vi "User_Manage.vi"() -> ()   [LabVIEW 2020]
panel:
  in  "User List":i32(listbox)
  # "用户管理"
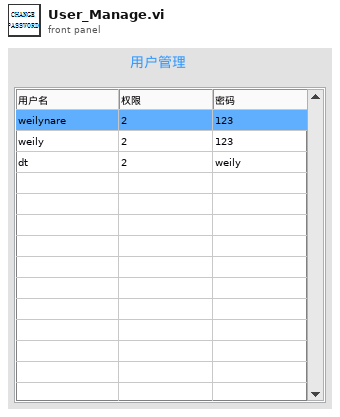
[diagram p1: front panel]
types:
  T1 = typedef "LVRowAndColumnTypeDef.ctl" = cluster{"Row":i32, "Column":i32}
  T2 = typedef "LVPoint32TypeDef.ctl" = cluster{"Horizontal":i32, "Vertical":i32}
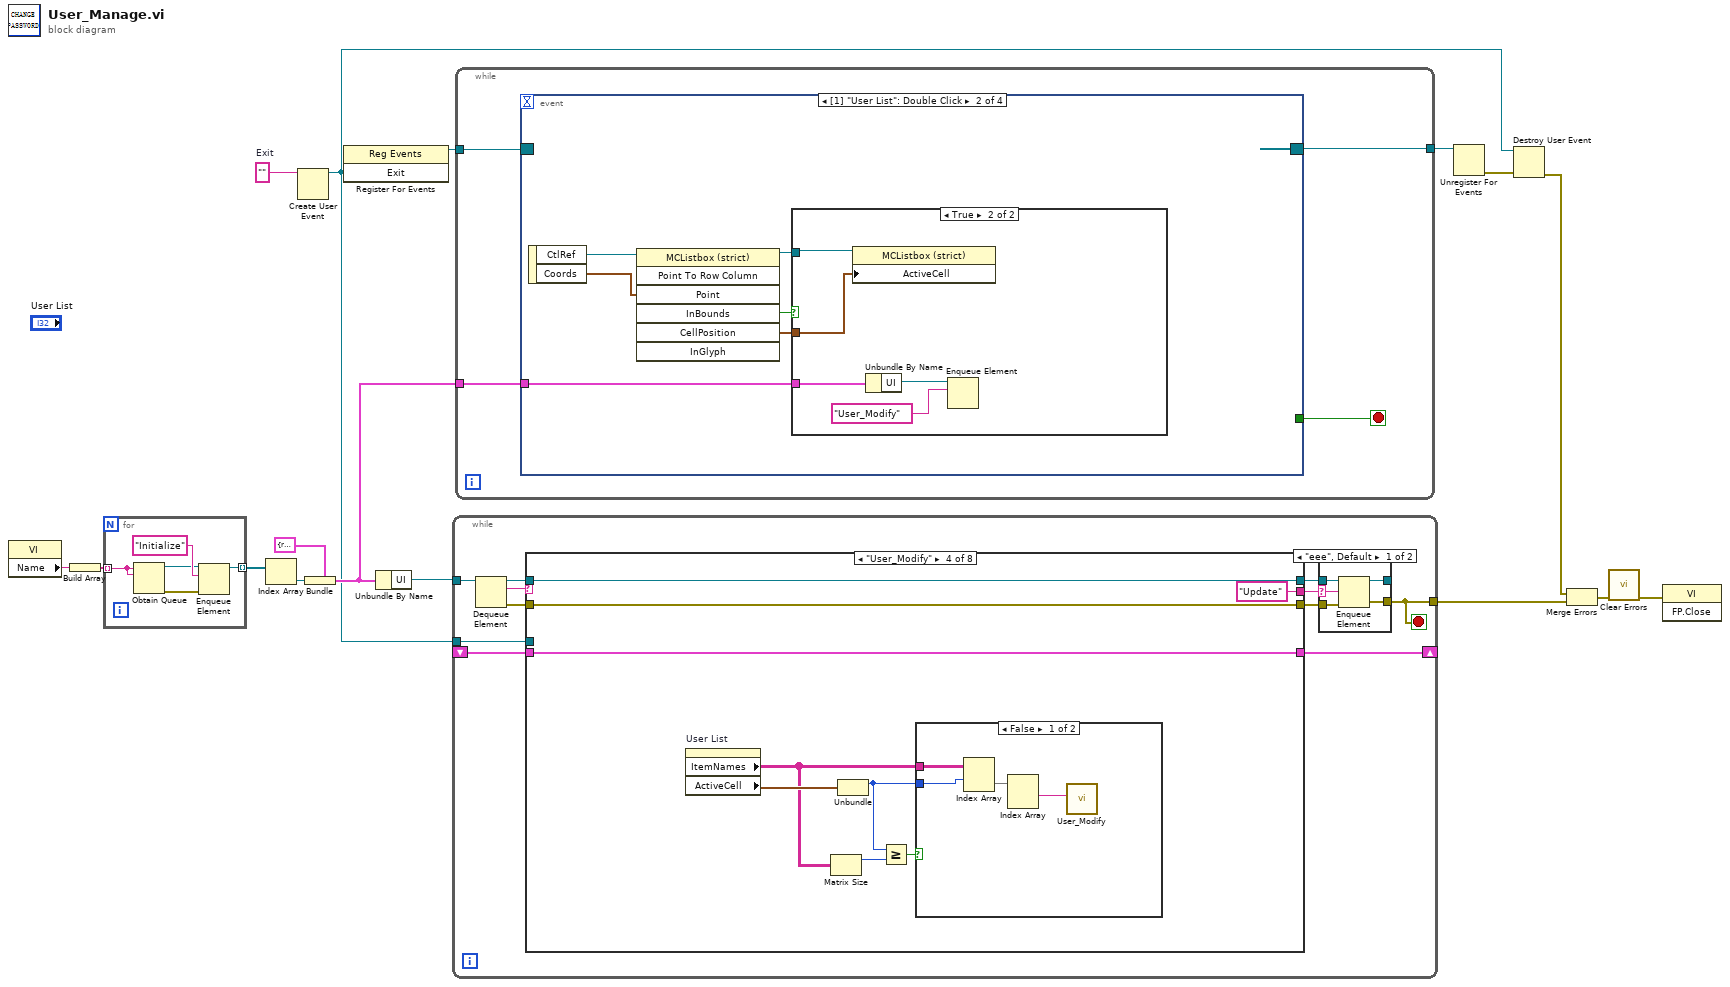
[diagram p0: block diagram]
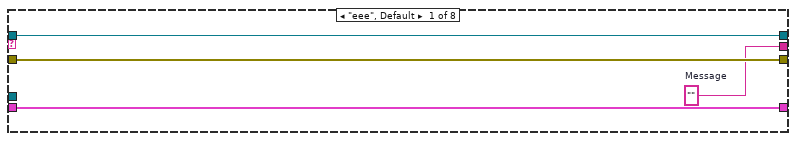
[diagram p3: hidden frame]
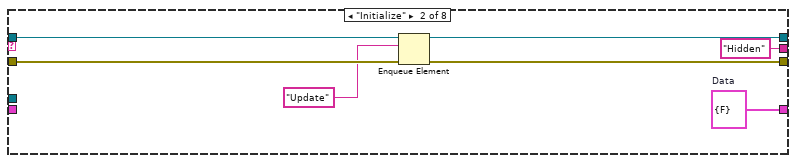
[diagram p4: hidden frame]
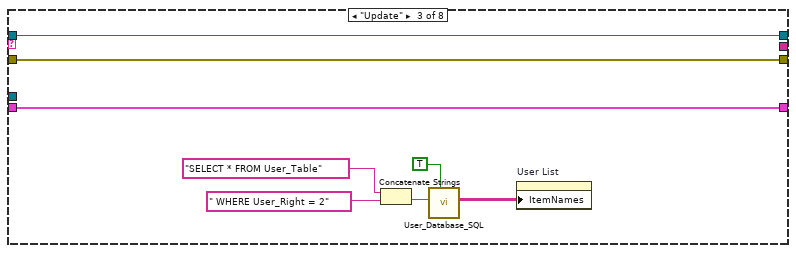
[diagram p5: hidden frame]
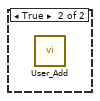
[diagram p6: hidden frame]
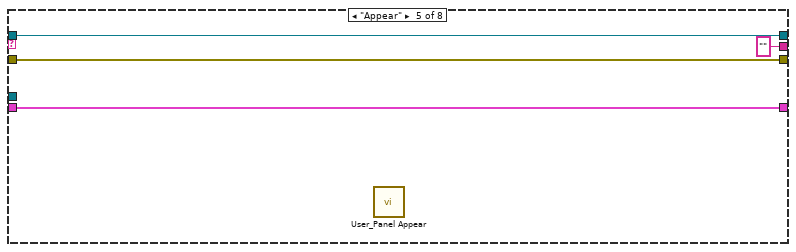
[diagram p7: hidden frame]
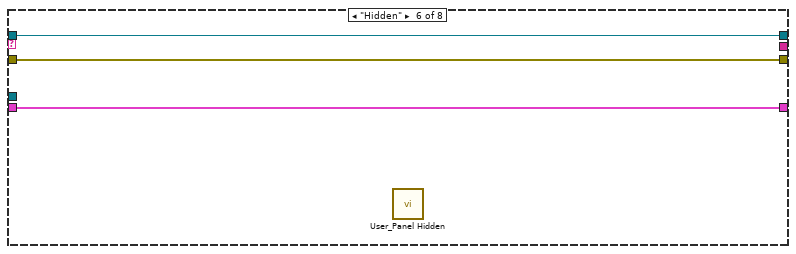
[diagram p8: hidden frame]
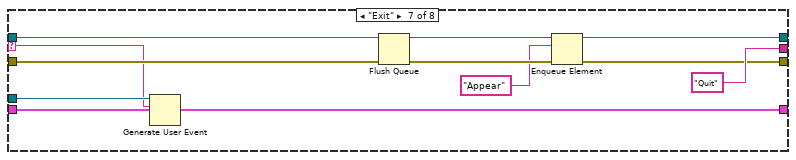
[diagram p9: hidden frame]
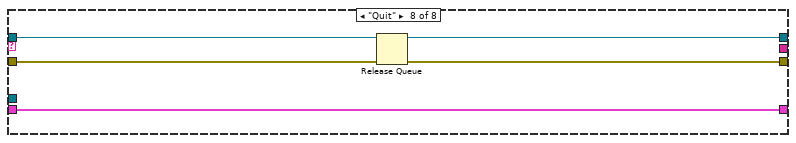
[diagram p10: hidden frame]
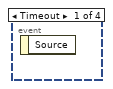
[diagram p11: hidden frame]
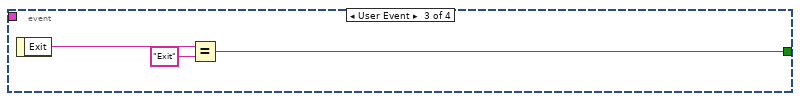
[diagram p13: hidden frame]
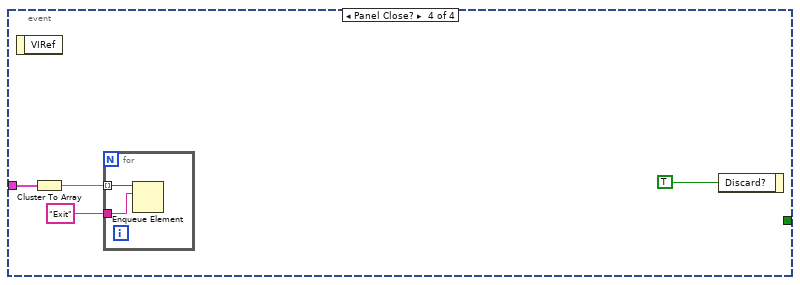
[diagram p14: hidden frame]
diagram:
  w2 = ""  # Exit
  n1 = property class="VI"() -> ("Name"=w12:string)  [unwired: 2 in, 2 out]
  n2 = Build Array(w12) -> (w13:string[])
  n3 = for {
    tunnel: w13 -> [w17] mode=indexing
    tunnel: [w18] -> w7 mode=indexing
    n4 = Obtain Queue(name (unnamed)=w17, element data type=w17) -> (queue out=w20:refnum<queue>, error out=w19:errorcluster)  [unwired: 3 in, 1 out]
    n5 = Enqueue Element(queue=w20, element="Initialize" ("元素"), error in (no error)=w19) -> (queue out=w18:refnum<queue>)  [unwired: 1 in, 2 out]
  }
  n6 = Index Array(array=w7) -> (element=w10:refnum<queue>)  [unwired: 1 in]
  n7 = Create User Event(user event datatype=w2) -> (user event=w6:refnum<user-event>)  [unwired: 1 in, 1 out]
  n8 = Bundle(cluster=cluster{"UI":refnum<queue>} {"UI"=refnum}, "UI"=w10) -> (w11:cluster{"UI":refnum<queue>})
  n9 = register-events(w6) -> (reference out=w3:refnum<event-registration>)  [unwired: 2 in, 1 out]
  n10 = Unbundle By Name(w11) -> ("UI"=w8:refnum<queue>)
  n11 = while {
    tunnel: w8 -> [w32]
    tunnel: [w22] -> w15
    shift-right: [w26] -> _
    shift-left: _ -> [w25]
    tunnel: w6 -> [w24]
    stop <- w22 stop-if-true
    n12 = Dequeue Element(queue=w32) -> (queue out=w31:refnum<queue>, element=w23:string, error out=w28:errorcluster)  [unwired: 2 in, 1 out]
    n13 = case shown="\"User_Modify\"" w23 {
      selector: w23 -> [_ _ _ _ _ _ w84 _]
      tunnel: w31 -> [w43 w48 w58 w67 w75 w78 w87 w93]
      tunnel: [w43 w47 w58 w67 w75 w78 w80 w93] -> w30
      tunnel: [w42 w45 w57 w66 w74 w77 w81 w90] -> w29
      tunnel: w28 -> [w42 w46 w57 w66 w74 w77 w86 w92]
      tunnel: [w41 "Hidden" ("Message") _ "Update" ("Message") "" ("Message") _ "Quit" ("Message") _] -> w27
      tunnel: [w40 w50 w56 w65 w73 w76 w89 w91] -> w26
      tunnel: w25 -> [w40 _ w56 w65 w73 w76 w89 w91]
      tunnel: w24 -> [_ _ _ _ _ _ w85 _]
      frame "eee", Default {
        w41 = ""  # Message
      }
      frame "Initialize" {
        w50 = cluster{"Data":bool} {"Data"=FALSE}  # Data
        n14 = Enqueue Element(queue=w48, element="Update" ("Message"), error in (no error)=w46) -> (queue out=w47:refnum<queue>, error out=w45:errorcluster)  [unwired: 1 in, 1 out]
      }
      frame "Update" {
        n15 = Concatenate Strings("SELECT * FROM User_Table" ("SQL query"), " WHERE User_Right = 2" ("SQL query")) -> (w53:string)
        n16 = call "User_Database_SQL.vi"("Get Record"=TRUE, "SQL query"=w53) -> ("Record"=w52:string[][])  [unwired: 7 in, 2 out]
        n17 = property on="User List" class="MCListbox (strict)"("ItemNames"=w52) -> ()  [unwired: 2 in, 2 out]
      }
      frame "User_Modify" {
        n18 = property on="User List" class="MCListbox (strict)"() -> ("ItemNames"=w62:string[][], "ActiveCell"=w63:T1)  [unwired: 2 in, 2 out]
        n19 = Matrix Size(0:w62) -> (1:w60:i32)  [unwired: 1 out]
        n20 = Unbundle(w63) -> ("Row"=w61:i32)  [unwired: 1 out]
        n21 = Greater Or Equal?(x=w61, y=w60) -> (x >= y?=w59:bool)
        n22 = case shown="False" w59 {
          tunnel: w62 -> [w69 _]
          tunnel: w61 -> [w68 _]
          frame False {
            n23 = Index Array(array=w69, index (row)=w68) -> (element=w71:string[])  [unwired: 1 in]
            n24 = Index Array(array=w71) -> (element #1=w70:string)  [unwired: 2 in, 1 out]
            n25 = call "User_Modify.vi"("User_Name"=w70) -> ()  [unwired: 11 in]
          }
          frame True {
            n26 = call "User_Add.vi"() -> ()  [unwired: 11 in, 1 out]
          }
        }
      }
      frame "Appear" {
        n27 = call "User_Panel Appear.vi"() -> ()  [unwired: 11 in, 1 out]
      }
      frame "Hidden" {
        n28 = call "User_Panel Hidden.vi"() -> ()  [unwired: 11 in, 1 out]
      }
      frame "Exit" {
        n29 = Generate User Event(user event=w85, event data cluster=w84) -> ()  [unwired: 2 in, 2 out]
        n30 = Flush Queue(queue=w87, error in (no error)=w86) -> (queue out=w83:refnum<queue>, error out=w82:errorcluster)  [unwired: 1 out]
        n31 = Enqueue Element(queue=w83, element="Appear" ("元素"), error in (no error)=w82) -> (queue out=w80:refnum<queue>, error out=w81:errorcluster)  [unwired: 1 in, 1 out]
      }
      frame "Quit" {
        n32 = Release Queue(queue=w93, error in (no error)=w92) -> (error out=w90:errorcluster)  [unwired: 1 in, 2 out]
      }
    }
    n33 = case shown="\"eee\", Default" w27 {
      selector: w27 -> [w33 _]
      tunnel: w30 -> [w37 w39]
      tunnel: w29 -> [w36 w38]
      tunnel: [w35 w38] -> w22
      tunnel: [w34 w39] -> _
      frame "eee", Default {
        n34 = Enqueue Element(queue=w37, element=w33, error in (no error)=w36) -> (queue out=w34:refnum<queue>, error out=w35:errorcluster)  [unwired: 1 in, 1 out]
      }
      frame "" {
      }
    }
  }
  n35 = while {
    tunnel: w3 -> [w96]
    tunnel: [w95] -> w5
    tunnel: w11 -> [w94]
    stop <- w97 stop-if-true
    n36 = event shown="[1] \"User List\": Double Click" {
      selector: w96 -> [_ _ _ _]
      dyn-events: [_ _ _ _] -> w95
      timeout: _ -> [_ _ _ _]
      tunnel: [_ _ w110 _] -> w97
      tunnel: w94 -> [_ w98 _ w114]
      event Timeout {
        n37 = event-data() -> ()  [unwired: 1 in, 1 out]
      }
      event "User List": Double Click {
        n38 = event-data() -> ("CtlRef"=w103:refnum<vi>, "Coords"=w102:T2)  [unwired: 1 in]
        n39 = invoke class="MCListbox (strict)" method="Point To Row Column"(reference=w103, "Point"=w102) -> (reference out=w99:refnum<vi>, "InBounds"=w101:bool, "CellPosition"=w100:T1)  [unwired: 5 in, 4 out]
        n40 = case shown="True" w101 {
          tunnel: w100 -> [_ w107]
          tunnel: w99 -> [_ w108]
          tunnel: w98 -> [_ w106]
          frame False {
          }
          frame True {
            n41 = property class="MCListbox (strict)"(reference=w108, "ActiveCell"=w107) -> ()  [unwired: 1 in, 2 out]
            n42 = Unbundle By Name(w106) -> ("UI"=w105:refnum<queue>)
            n43 = Enqueue Element(queue=w105, element="User_Modify" ("元素")) -> ()  [unwired: 2 in, 3 out]
          }
        }
      }
      event User Event {
        n44 = event-data() -> ("Exit"=w111:string)  [unwired: 1 in]
        n45 = Equal?(x=w111, y="Exit") -> (x = y?=w110:bool)
      }
      event Panel Close? {
        n46 = event-data() -> ()  [unwired: 1 in, 1 out]
        n47 = Cluster To Array(cluster=w114) -> (array=w113:refnum<queue>[])
        n48 = for {
          tunnel: w113 -> [w117] mode=indexing
          tunnel: "Exit" ("元素") -> [w116]
          n49 = Enqueue Element(queue=w117, element=w116) -> ()  [unwired: 2 in, 3 out]
        }
        n50 = event-data("Discard?"=TRUE ("放弃？")) -> ()  [unwired: 1 in, 1 out]
      }
    }
  }
  n51 = Unregister For Events(event registration refnum=w5) -> (error out=w4:errorcluster)  [unwired: 1 in]
  n52 = Destroy User Event(user event=w6, error in=w4) -> (error out=w14:errorcluster)
  n53 = Merge Errors(w14, w15) -> (w16:errorcluster)
  n54 = call <vilib>:"Clear Errors.vi"("error in (no error)"=w16) -> ("error out"=w1:errorcluster)  [unwired: 5 in, 1 out]
  n55 = invoke class="VI" method="FP.Close"(error in=w1) -> ()  [unwired: 2 in, 3 out]
